vi "Restart_Compressor.vi"(0 "Restart_Compressor":bool) -> ()   [LabVIEW 2018]
uses:
  Global_Variables/Refnum_Names.vi
  <vilib>/Rock Robotics/WPI/Utilities/WPI_GetSetVariantRefNum.vi
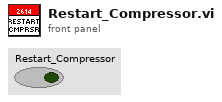
[diagram p1: front panel]
types:
  T1 = typedef "WPI_CompressorDevRef.ctl" = cluster{"DevStatus":errorcluster, "Pneumatics Control Module":u8}
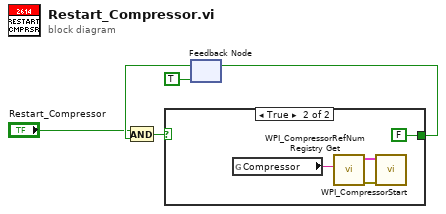
[diagram p0: block diagram]
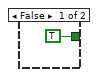
[diagram p2: hidden frame]
diagram:
  n1 = feedback #1(TRUE) -> (w3:bool)
  n2 = And(x="Restart_Compressor", y=w3) -> (x .and. y?=w2:bool)
  n3 = case shown="True" w2 {
    tunnel: [TRUE FALSE] -> w5
    frame False {
    }
    frame True {
      n4 = global read "Refnum_Names.vi" "Compressor"() -> (w7:string)
      n5 = call <vilib>:"WPI_CompressorRefNum Registry Get.vi"("refnum name"=w7) -> ("error out"=w9:errorcluster, "CompressorDevRef"=w10:T1)  [unwired: 9 in]
      n6 = call <vilib>:"WPI_CompressorStart.vi"("error in (no error)"=w9, "CompressorDevRef"=w10) -> ()  [unwired: 8 in, 2 out]
    }
  }
  n7 = feedback-in #1(w5) -> ()
